vi "CANOpen Refresh Device Node.vi"(8 "error in (no error)":errorcluster, 11 "Node Ptr":u64 format="%.0x") -> (0 "error out":errorcluster)   [LabVIEW 2021, in "CANOpen Addon System Explorer.lvlib"]
uses:
  CANOpen Addon System Explorer.lvlib
panel:
  in  "Tag":string
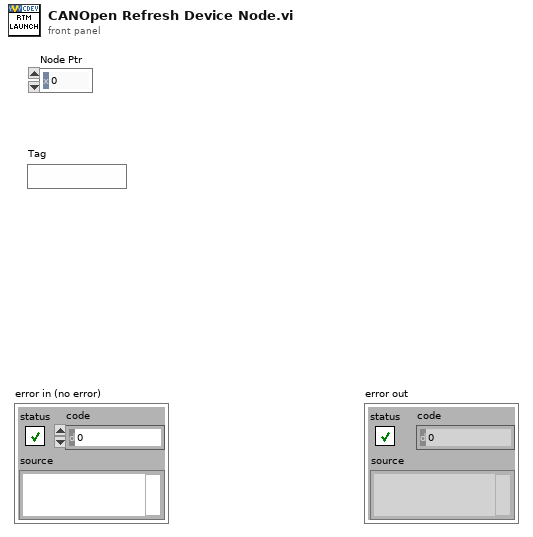
[diagram p1: front panel]
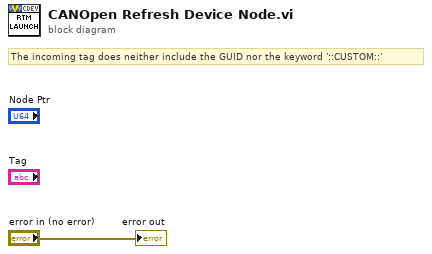
[diagram p0: block diagram]
diagram:
  # "The incoming tag does neither include the GUID nor the keyword '::CUSTOM::'"
  "error out" <- "error in (no error)"
